vi "golpi_mpc_start_octave_low_level.vi"(7 "don't query version (true)":bool=TRUE, 8 "error in":errorcluster, 10 "allow octave start (true)":bool=TRUE, 11 "golpi session in":T1={"GOLPI ref"={"pipe handle"={"lv_proc.dll file path"=path "", "process instance handle"=[], "debug mode"=FALSE, "debug data"=[]}, "fast read timeout [ms]"=500, "fast read settle time [ms]"=10, "fast read to multiple [ms]"=1, "max elements per input line"=100, "slow read timeout [ms]"=5000, "stdin double format specifier"="%_16e", "max elements per stdout output column"=100, "console mode bitstream"=FALSE, "bitstream first read timeout [ms]"=1000, "bitstream read timeout [ms]"=50, "struct transfer possible"=FALSE, "matlab mode"=FALSE}, "idn str"="", "octave path"=path "C:/Octave364/Octave3.6.4_gcc4.6.2/bin", "work path"=path "C:/Octave364/Octave3.6.4_gcc4.6.2/bin", "start timeout [ms]"=15000, "clr cache"=FALSE, "console"=FALSE, "binary"=FALSE, "semaphore"=refnum, "initial command"="", "exit command"="", "matlab"=FALSE}) -> (0 "error out":errorcluster, 1 "octave started (was closed)":bool, 2 "GNU Octave version":string, 3 "golpi session out":T1={"GOLPI ref"={"pipe handle"={"lv_proc.dll file path"=path "", "process instance handle"=[], "debug mode"=FALSE, "debug data"=[]}, "fast read timeout [ms]"=500, "fast read settle time [ms]"=10, "fast read to multiple [ms]"=1, "max elements per input line"=100, "slow read timeout [ms]"=5000, "stdin double format specifier"="%_16e", "max elements per stdout output column"=100, "console mode bitstream"=FALSE, "bitstream first read timeout [ms]"=1000, "bitstream read timeout [ms]"=50, "struct transfer possible"=FALSE, "matlab mode"=FALSE}, "idn str"="", "octave path"=path "C:/Octave364/Octave3.6.4_gcc4.6.2/bin", "work path"=path "C:/Octave364/Octave3.6.4_gcc4.6.2/bin", "start timeout [ms]"=15000, "clr cache"=FALSE, "console"=FALSE, "binary"=FALSE, "semaphore"=refnum, "initial command"="", "exit command"="", "matlab"=FALSE})   [LabVIEW 2018, in "GOLPI Multi Process.lvlib"]
doc: "Multi-process GOLPI internal function: Starts GOLPI (Octave) or just queries version unless it is not inhibited.\n\nIf start allowed and Octave is not running it will start it with options defined in GOLPI session. After the startup it will eventually execute initial command defined in the GOLPI session (usafull for instance for initial path setup, restoring environment variables or whatever...). \n\nIf start not allowef and not running it does nothing.\n\nIf already started and version query is not inhibited it will return version string. Otherwise it does nothing."
uses:
  GOLPI Multi Process.lvlib
  golpi_session.ctl
  GOLPI Library.lvlibp/Public/GOLPI reference Type Def.ctl
  GOLPI Library.lvlibp/LV Process source distribution/Pipe Handle.ctl
  GOLPI Library.lvlibp/Private/Get Variable - polymorph parts/Get String.vi
  GOLPI Library.lvlibp
  varilib/varilib.lvlib
  GOLPI Library.lvlibp/LV Process source distribution/LV Process library.lvlib
panel:
  out "not running?":bool
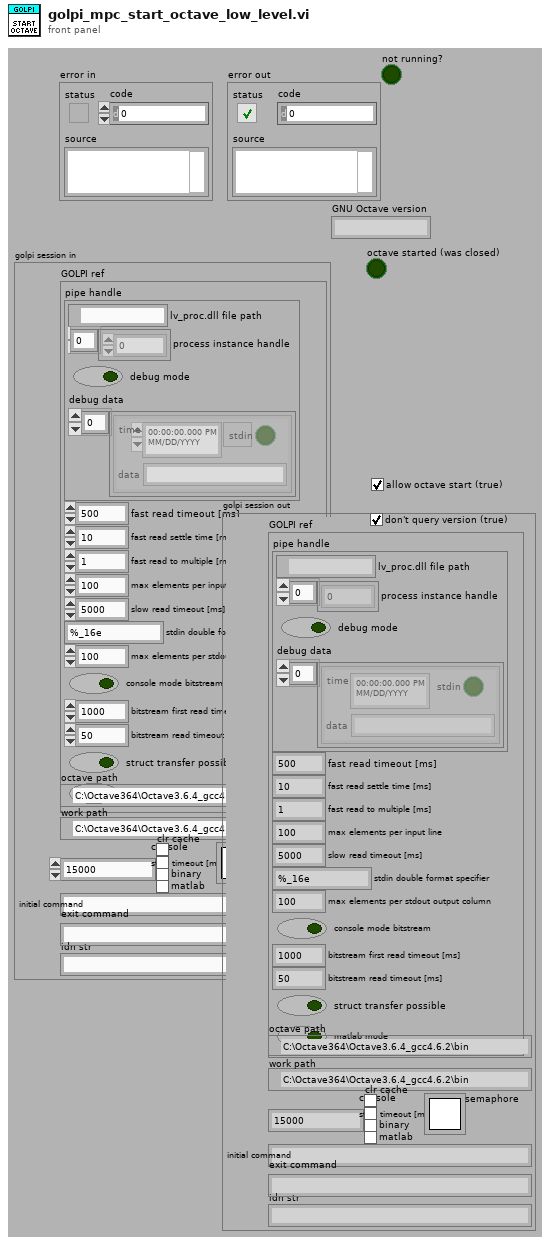
[diagram p1: front panel]
types:
  T1 = typedef "GOLPI Multi Process.lvlib/golpi_session.ctl" = cluster{"GOLPI ref":T2, "idn str":string, "octave path":path, "work path":path, "start timeout [ms]":u32, "clr cache":bool, "console":bool, "binary":bool, "semaphore":T4, "initial command":string, "exit command":string, "matlab":bool}
  T2 = typedef "GOLPI Library.lvlibp/GOLPI reference Type Def.ctl" = cluster{"pipe handle":T3, "fast read timeout [ms]":u32, "fast read settle time [ms]":u32, "fast read to multiple [ms]":u32, "max elements per input line":u32, "slow read timeout [ms]":u32, "stdin double format specifier":string, "max elements per stdout output column":u32, "console mode bitstream":bool, "bitstream first read timeout [ms]":u32, "bitstream read timeout [ms]":u32, "struct transfer possible":bool, "matlab mode":bool}
  T3 = typedef "GOLPI Library.lvlibp/LV Process library.lvlib/Pipe Handle.ctl" = cluster{"lv_proc.dll file path":path, "process instance handle":u32[], "debug mode":bool, "debug data":cluster{"time":timestamp, "stdin":bool, "data":string}[]}
  T4 = typedef "Semaphore RefNum" = refnum<k1>
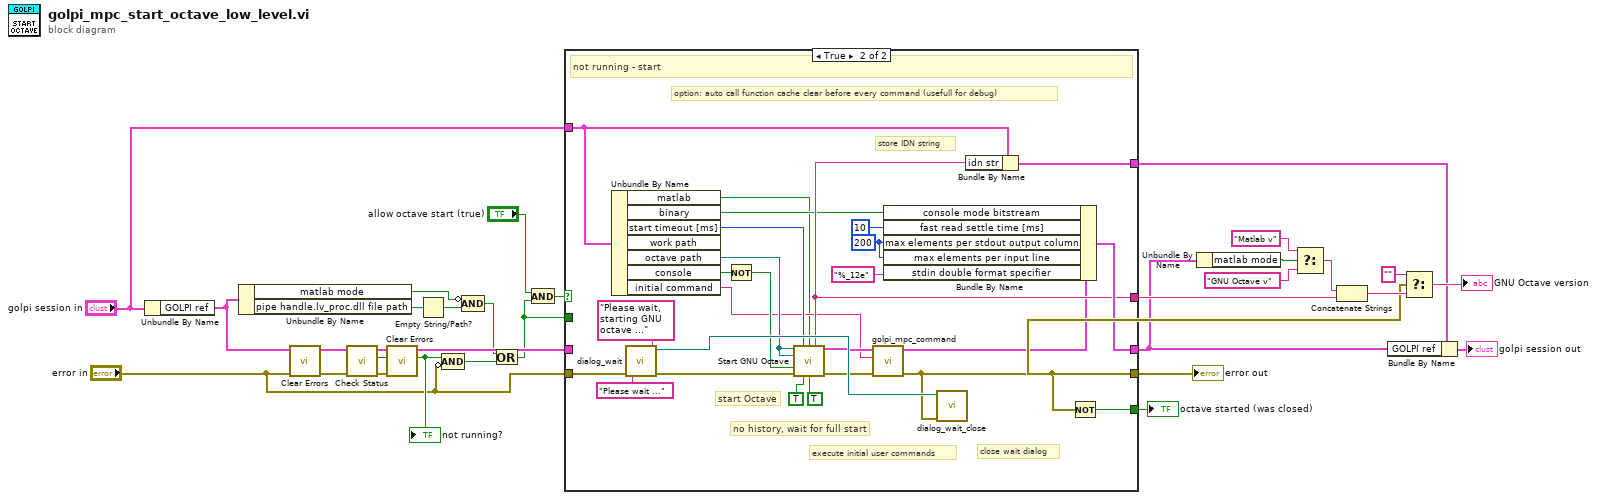
[diagram p0: block diagram]
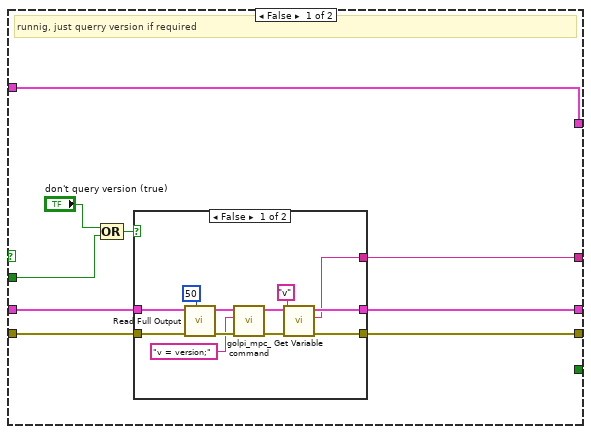
[diagram p2: hidden frame]
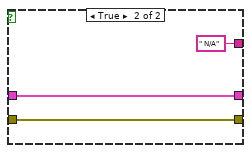
[diagram p3: hidden frame]
diagram:
  n1 = Unbundle By Name("golpi session in") -> ("GOLPI ref"=w17:T2)
  n2 = Unbundle By Name(w17) -> ("matlab mode"=w2:bool, "pipe handle.lv_proc.dll file path"=w26:path)
  n3 = call <vilib>:"Clear Errors.vi"("error in (no error)"="error in") -> ("error out"=w24:errorcluster)  [unwired: 5 in, 1 out]
  n4 = call "Check Status.vi"("error in"=w24, "GOLPI ref. in"=w17) -> ("error out"=w23:errorcluster, "exited?"=w28:bool, "GOLPI ref. out"=w27:T2)  [unwired: 7 in]
  "not running?" <- w28
  n5 = call <vilib>:"Clear Errors.vi"("error in (no error)"=w23) -> ()  [unwired: 5 in, 2 out]
  n6 = Empty String/Path?(string/path=w26) -> (empty?=w3:bool)
  n7 = Compound Arithmetic op=AND(w28, invert "error in") -> (w25:bool)
  n8 = Compound Arithmetic op=AND(invert w2, w3) -> (w1:bool)
  n9 = Or(x=w1, y=w25) -> (x .or. y?=w11:bool)
  n10 = And(x="allow octave start (true)", y=w11) -> (x .and. y?=w13:bool)
  n11 = case shown="True" w13 {
    tunnel: "error in" -> [w37 w77]
    tunnel: w27 -> [w36 _]
    tunnel: [w35 w57] -> w15
    tunnel: [w34 w68] -> w8
    tunnel: [w33 w61] -> w19
    tunnel: "golpi session in" -> [w29 w63]
    tunnel: [_ w64] -> w14
    tunnel: w11 -> [w30 _]
    tunnel: [w29 w62] -> w9
    frame False {
      # "runnig, just querry version if required"
      n12 = Compound Arithmetic op=OR("don't query version (true)", w30) -> (w31:bool)
      n13 = case shown="False" w31 {
        tunnel: w37 -> [w48 w52]
        tunnel: w36 -> [w47 w51]
        tunnel: [w42 w52] -> w35
        tunnel: [w40 w51] -> w34
        tunnel: [w38 " N/A" ("value")] -> w33
        frame False {
          n14 = call "Read Full Output.vi"("timeout [ms]"=u32 50, "error in"=w48, "GOLPI ref. in"=w47) -> ("error out"=w46:errorcluster, "GOLPI ref. out"=w45:T2)  [unwired: 5 in, 2 out]
          n15 = call "golpi_mpc_command.vi"("error in"=w46, "command"="v = version;", "GOLPI ref in"=w45) -> ("error out"=w43:errorcluster, "GOLPI ref. out"=w41:T2)  [unwired: 6 in, 1 out]
          n16 = call-poly "Get Variable.vi"("error in"=w43, "variable name"="v", "GOLPI ref. in"=w41) -> ("error out"=w42:errorcluster, "value"=w38:string, "GOLPI ref. out"=w40:T2)  [unwired: 6 in]
        }
        frame True {
        }
      }
    }
    frame True {
      w65 = u32 200 ("max elements per stdout output column")
      # "close wait dialog"
      # "option: auto call function cache clear before every command (usefull for debug)"
      # "store IDN string"
      # "execute initial user commands"
      # "no history, wait for full start"
      # "start Octave"
      # "not running - start"
      n17 = Unbundle By Name(w63) -> ("matlab"=w53:bool, "binary"=w55:bool, "start timeout [ms]"=w71:u32, "octave path"=w69:path, "console"=w70:bool, "initial command"=w58:string)  [unwired: 1 out]
      n18 = call "dialog_wait.vi"("error in"=w77, "title string"="Please wait ..." ("title"), "message string"="Please wait, starting GNU octave ..." ("msg")) -> ("error out"=w72:errorcluster, "reference out"=w74:refnum<vi>)  [unwired: 7 in]
      n19 = Not(x=w70) -> (.not. x?=w73:bool)
      n20 = call "Start GNU Octave.vi"("working directory"=w69, "full start timeout [ms] (20000)"=w71, "Matlab script mode (F)"=w53, "octave exe file or directory"=w69, "hide debug console (T)"=w73, "error in"=w72, "wait for full start (T)"=TRUE ("Wait for full GNU Octave start"), "disable history (T)"=TRUE) -> ("GNU Octave version"=w61:string, "GOLPI ref. out"=w59:T2, "error out"=w60:errorcluster)  [unwired: 4 in, 1 out]
      n21 = call "golpi_mpc_command.vi"("error in"=w60, "command"=w58, "GOLPI ref in"=w59) -> ("error out"=w57:errorcluster, "GOLPI ref. out"=w56:T2)  [unwired: 6 in, 1 out]
      n22 = Bundle By Name(cluster=w56, "console mode bitstream"=w55, "fast read settle time [ms]"=u32 10, "max elements per stdout output column"=w65, "max elements per input line"=w65, "stdin double format specifier"="%_12e") -> (w68:T2)
      n23 = call "dialog_wait_close.vi"("error in"=w57, "async vi ref"=w74) -> ()  [unwired: 2 in]
      n24 = Bundle By Name(cluster=w63, "idn str"=w61) -> (w62:T1)
      n25 = Not(x=w57) -> (.not. x?=w64:bool)
    }
  }
  "error out" <- w15
  "octave started (was closed)" <- w14
  n26 = Unbundle By Name(w8) -> ("matlab mode"=w7:bool)
  n27 = Select(t="Matlab v" ("string"), s=w7, f="GNU Octave v" ("string")) -> (s? t:f=w4:string)
  n28 = Concatenate Strings(w4, w19) -> (w22:string)
  n29 = Bundle By Name(cluster=w9, "GOLPI ref"=w8) -> (→"golpi session out":T1)
  n30 = Select(t="", s=w15, f=w22) -> (s? t:f=→"GNU Octave version":string)
